vi "RT Engine.vi"(8 "Error In":errorcluster) -> ()   [LabVIEW 2013]
uses:
  <vilib>/NI/STM/TCP/TCP Connection Info.ctl
  <vilib>/NI/STM/SubVIs/MetaDataElement.ctl
  <vilib>/NI/STM/Connection Manager/TCP/TCP Connection Method.ctl
  PC/Event Mode.ctl
  <vilib>/NI/STM/Connection Manager/TCP/TCP Connection Properties.ctl
  <vilib>/NI/STM/TCP/TCP Read Options.ctl
  PC/PCsend RTrecv CMD.ctl
  TypeDef/TCP Cluster.ctl
  <vilib>/NI/STM/TCP/Write Meta Data (TCP Ref).vi
  <vilib>/NI/STM/TCP/Write Meta Data (TCP Clst).vi
  <vilib>/NI/STM/TCP/Read Message (TCP).vi
  <vilib>/NI/STM/TCP/Write Message (TCP).vi
  <vilib>/NI/STM/NI STM.lvlib
panel:
  out "conn?":bool
  out "SEND conn":T1
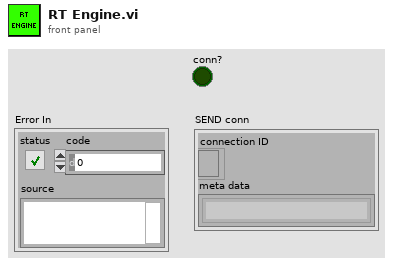
[diagram p1: front panel]
types:
  T1 = typedef "NI STM.lvlib/TCP Connection Info.ctl" = cluster{"connection ID":refnum<k5>, "meta data":T2[]}
  T2 = typedef "NI STM.lvlib/MetaDataElement.ctl" = string
  T3 = typedef "Event Mode.ctl" = enum16{"Init", "Get", "Set", "Destroy"}
  T4 = typedef "NI STM.lvlib/TCP Connection Method.ctl" = enum16{"Initialize", "Add Connection", "Set Properties", "Get Connection(s)", "Remove Connection", "Remove All Connections", "Get Connection Count"}
  T5 = typedef "NI STM.lvlib/TCP Connection Properties.ctl" = cluster{"Name":string, "Address":string, "Custom":string}
  T6 = typedef "NI STM.lvlib/TCP Read Options.ctl" = cluster{"ignore timeout error":bool, "timeout ms (1000)":i32}
  T7 = typedef "PCsend RTrecv CMD.ctl" = enum16{"ConnSettings", "Connect", "CMD", "Controller", "PSenable", "ReqCalDate", "Tolerances", "Stable Trigger", "Stop", "VPLimits", "NeedleValve", "SpeedWindow", "FreezeCmdPID", "LoadFPGA"}
  T8 = typedef "TCP Cluster.ctl" = cluster{"Command":string, "FlattenedData":string}
  T9 = typedef "RTsend PCrecv CMD.ctl" = enum16{"Data", "Connected?", "CalFileDate"}
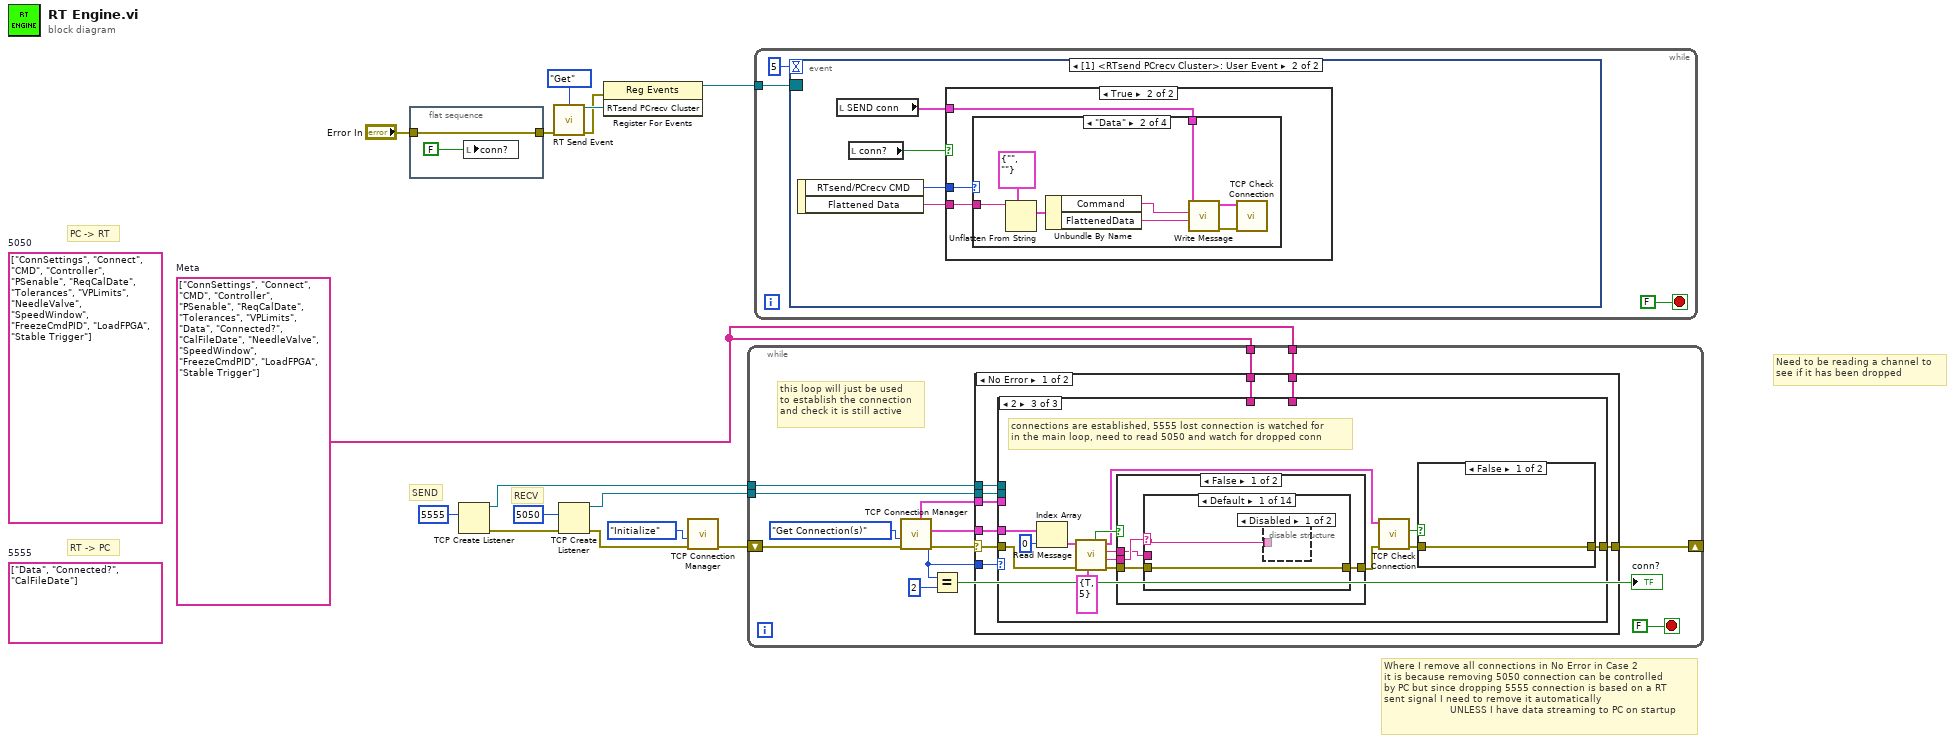
[diagram p0: block diagram]
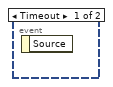
[diagram p2: hidden frame]
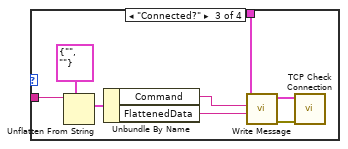
[diagram p5: hidden frame]
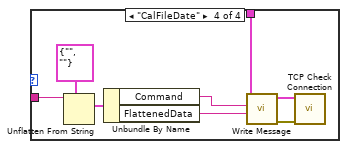
[diagram p6: hidden frame]
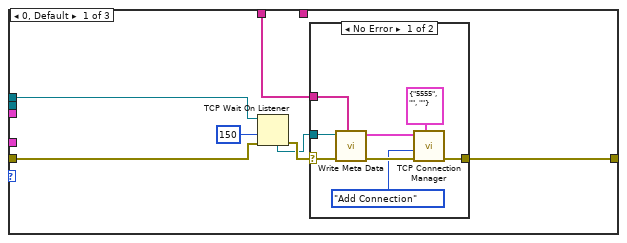
[diagram p7: hidden frame]
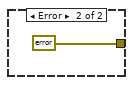
[diagram p8: hidden frame]
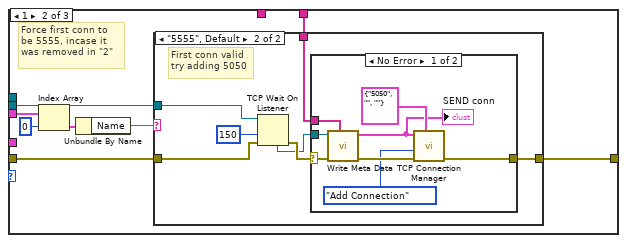
[diagram p9: hidden frame]
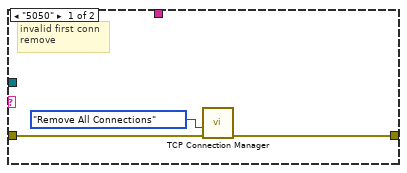
[diagram p10: hidden frame]
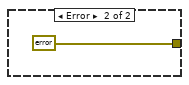
[diagram p11: hidden frame]
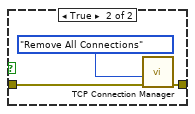
[diagram p12: hidden frame]
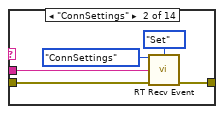
[diagram p14: hidden frame]
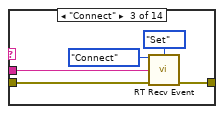
[diagram p15: hidden frame]
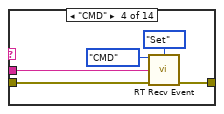
[diagram p16: hidden frame]
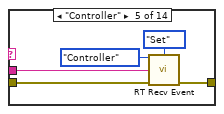
[diagram p17: hidden frame]
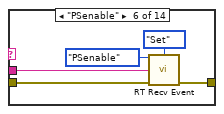
[diagram p18: hidden frame]
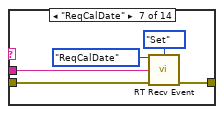
[diagram p19: hidden frame]
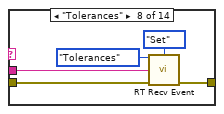
[diagram p20: hidden frame]
diagram:
  w1 = T2[] ["ConnSettings", "Connect", "CMD", "Controller", "PSenable", "ReqCalDate", "Tolerances", "VPLimits", "Data", "Connected?", "CalFileDate", "NeedleValve", "SpeedWindow", "FreezeCmdPID", "LoadFPGA", "Stable Trigger"]  # Meta
  (unwired) T2[] ["Data", "Connected?", "CalFileDate"]  # 5555
  (unwired) T2[] ["ConnSettings", "Connect", "CMD", "Controller", "PSenable", "ReqCalDate", "Tolerances", "VPLimits", "NeedleValve", "SpeedWindow", "FreezeCmdPID", "LoadFPGA", "Stable Trigger"]  # 5050
  # "PC -> RT"
  # "RT -> PC"
  # "Where I remove all connections in No Error in Case 2\nit is because removing 5050 connection can be controlled\nby PC but since dropping 5555 connection is based on a RT\nsent signal I need to remove it automatically\n                      UNLESS I have data streaming to PC on startup"
  # "Need to be reading a channel to\nsee if it has been dropped"
  # "SEND"
  # "RECV"
  n1 = flat-sequence {
    tunnel: "Error In" -> [w17]
    tunnel: [w17] -> w8
    frame #0 {
      n2 = local write "conn?"(FALSE ("stop")) -> ()
    }
  }
  n3 = TCP Create Listener(10:u16 5555 ("port")) -> (0:w6:errorcluster, 3:w5:refnum<k5>)  [unwired: 4 in, 1 out]
  n4 = call "RT Send Event.vi"("Mode"=Event_Mode."Get", "Error In"=w8) -> ("RTsend PCrecv Cluster"=w12:refnum<user-event>, "Error Out"=w11:errorcluster)  [unwired: 12 in]
  n5 = TCP Create Listener(8:w6, 10:u16 5050 ("port")) -> (0:w15:errorcluster, 3:w4:refnum<k5>)  [unwired: 3 in, 1 out]
  n6 = register-events(error in=w11, w12) -> (reference out=w10:refnum<event-registration>)  [unwired: 1 in, 1 out]
  n7 = call <vilib>:"TCP Connection Manager.vi"("error in"=w15, "method"=TCP_Connection_Method."Initialize") -> ("error out"=w13:errorcluster)  [unwired: 4 in, 5 out]
  n8 = while {
    shift-right: [w19] -> _
    shift-left: w13 -> [w31]
    tunnel: w1 -> [w28]
    tunnel: w5 -> [w25]
    tunnel: w4 -> [w24]
    tunnel: w1 -> [w18]
    stop <- FALSE stop-if-true
    # "this loop will just be used\nto establish the connection\nand check it is still active"
    n9 = call <vilib>:"TCP Connection Manager.vi"("error in"=w31, "method"=TCP_Connection_Method."Get Connection(s)") -> ("error out"=w29:errorcluster, "number of connections"=w21:i32, "all connections"=w23:T1[], "all properties"=w22:T5[])  [unwired: 4 in, 2 out]
    n10 = Equal?(x=w21, y=2) -> (x = y?=→"conn?":bool)
    n11 = case shown="No Error" w29 {
      selector: w29 -> [w40 _]
      tunnel: [w39 errorcluster {"status"=FALSE, "code"=0, "source"=""} ("t")] -> w19
      tunnel: w28 -> [w38 _]
      tunnel: w25 -> [w37 _]
      tunnel: w24 -> [w36 _]
      tunnel: w23 -> [w33 w176]
      tunnel: w22 -> [w34 _]
      tunnel: w21 -> [w35 _]
      tunnel: w18 -> [w32 _]
      frame No Error {
        n12 = case shown="2" w35 {
          tunnel: [w46 w64 w94] -> w39
          tunnel: w40 -> [w47 w57 w95]
          tunnel: w38 -> [_ w63 _]
          tunnel: w37 -> [w45 _ _]
          tunnel: w36 -> [_ w58 _]
          tunnel: w34 -> [_ w62 _]
          tunnel: w33 -> [_ _ w97]
          tunnel: w32 -> [w41 _ _]
          frame 0, Default {
            n13 = TCP Wait On Listener(8:w47, 9:150 ("timeout ms (wait forever: -1)"), 11:w45) -> (0:w43:errorcluster, 4:w42:refnum<k5>)  [unwired: 1 in, 3 out]
            n14 = case shown="No Error" w43 {
              selector: w43 -> [w55 _]
              tunnel: [w53 errorcluster {"status"=FALSE, "code"=0, "source"=""} ("error constant")] -> w46
              tunnel: w42 -> [w52 _]
              tunnel: w41 -> [w50 _]
              frame No Error {
                n15 = call-poly <vilib>:"Write Meta Data.vi"("meta data"=w50, "error in"=w55, "connection ID"=w52) -> ("error out"=w54:errorcluster, "connection info out"=w48:T1)  [unwired: 7 in]
                n16 = call <vilib>:"TCP Connection Manager.vi"("properties in"=T5 {"Name"="5555", "Address"="", "Custom"=""}, "error in"=w54, "method"=TCP_Connection_Method."Add Connection", "connection in"=w48) -> ("error out"=w53:errorcluster)  [unwired: 2 in, 5 out]
              }
              frame Error {
              }
            }
          }
          frame 1 {
            # "Force first conn to\nbe 5555, incase it\nwas removed in \"2\""
            n17 = Index Array(array=w62, index=0) -> (element=w61:T5)
            n18 = Unbundle By Name(w61) -> ("Name"=w59:string)
            n19 = case shown="\"5555\", Default" w59 {
              tunnel: [w65 w74] -> w64
              tunnel: w63 -> [_ w73]
              tunnel: w57 -> [w66 w69]
              tunnel: w58 -> [_ w68]
              frame "5050" {
                # "invalid first conn\nremove"
                n20 = call <vilib>:"TCP Connection Manager.vi"("error in"=w66, "method"=TCP_Connection_Method."Remove All Connections") -> ("error out"=w65:errorcluster)  [unwired: 4 in, 5 out]
              }
              frame "5555", Default {
                # "First conn valid\ntry adding 5050"
                n21 = TCP Wait On Listener(8:w69, 9:150 ("timeout ms (wait forever: -1)"), 11:w68) -> (0:w71:errorcluster, 4:w70:refnum<k5>)  [unwired: 1 in, 3 out]
                n22 = case shown="No Error" w71 {
                  selector: w71 -> [w82 _]
                  tunnel: [w80 errorcluster {"status"=FALSE, "code"=0, "source"=""} ("error constant")] -> w74
                  tunnel: w70 -> [w79 _]
                  tunnel: w73 -> [w77 _]
                  frame No Error {
                    n23 = call-poly <vilib>:"Write Meta Data.vi"("meta data"=w77, "error in"=w82, "connection ID"=w79) -> ("error out"=w81:errorcluster, "connection info out"=w75:T1)  [unwired: 7 in]
                    "SEND conn" <- w75
                    n24 = call <vilib>:"TCP Connection Manager.vi"("properties in"=T5 {"Name"="5050", "Address"="", "Custom"=""}, "error in"=w81, "method"=TCP_Connection_Method."Add Connection", "connection in"=w75) -> ("error out"=w80:errorcluster)  [unwired: 2 in, 5 out]
                  }
                  frame Error {
                  }
                }
              }
            }
          }
          frame 2 {
            # "connections are established, 5555 lost connection is watched for\nin the main loop, need to read 5050 and watch for dropped conn"
            n25 = Index Array(array=w97, index=0) -> (element=w93:T1)
            n26 = call-poly <vilib>:"Read Message.vi"("options"=T6 {"ignore timeout error"=TRUE, "timeout ms (1000)"=5}, "error in"=w95, "connection info in"=w93) -> ("error out"=w91:errorcluster, "name"=w90:T2, "data string"=w89:string, "connection info out"=w88:T1, "timed out?"=w92:bool)  [unwired: 3 in, 1 out]
            n27 = case shown="False" w92 {
              tunnel: w91 -> [w104 w173]
              tunnel: [w103 w173] -> w87
              tunnel: w90 -> [w105 _]
              tunnel: w89 -> [w102 _]
              frame False {
                n28 = case shown="Default" w105 {
                  selector: w105 -> [w106 _ _ _ _ _ _ _ _ _ _ _ _ _]
                  tunnel: w104 -> [w107 w111 w116 w121 w126 w131 w136 w141 w146 w151 w156 w161 w166 w171]
                  tunnel: [w107 w110 w114 w120 w125 w129 w135 w139 w144 w149 w154 w159 w164 w169] -> w103
                  tunnel: w102 -> [_ w109 w115 w119 w124 w130 w134 w140 w145 w150 w155 w160 w165 w170]
                  frame Default {
                    n29 = disable-structure shown="Disabled" {
                      disable-tunnel: w106 -> [_ _]
                      frame Disabled {
                      }
                      frame Enabled {
                      }
                    }
                  }
                  frame "ConnSettings" {
                    n30 = call "RT Recv Event.vi"("PCsend/RTrecv CMD"=PCsend_RTrecv_CMD."ConnSettings", "Mode"=Event_Mode."Set", "Flattened Data"=w109, "Error In"=w111) -> ("Error Out"=w110:errorcluster)  [unwired: 10 in, 1 out]
                  }
                  frame "Connect" {
                    n31 = call "RT Recv Event.vi"("PCsend/RTrecv CMD"=PCsend_RTrecv_CMD."Connect", "Mode"=Event_Mode."Set", "Flattened Data"=w115, "Error In"=w116) -> ("Error Out"=w114:errorcluster)  [unwired: 10 in, 1 out]
                  }
                  frame "CMD" {
                    n32 = call "RT Recv Event.vi"("PCsend/RTrecv CMD"=PCsend_RTrecv_CMD."CMD", "Mode"=Event_Mode."Set", "Flattened Data"=w119, "Error In"=w121) -> ("Error Out"=w120:errorcluster)  [unwired: 10 in, 1 out]
                  }
                  frame "Controller" {
                    n33 = call "RT Recv Event.vi"("PCsend/RTrecv CMD"=PCsend_RTrecv_CMD."Controller", "Mode"=Event_Mode."Set", "Flattened Data"=w124, "Error In"=w126) -> ("Error Out"=w125:errorcluster)  [unwired: 10 in, 1 out]
                  }
                  frame "PSenable" {
                    n34 = call "RT Recv Event.vi"("PCsend/RTrecv CMD"=PCsend_RTrecv_CMD."PSenable", "Mode"=Event_Mode."Set", "Flattened Data"=w130, "Error In"=w131) -> ("Error Out"=w129:errorcluster)  [unwired: 10 in, 1 out]
                  }
                  frame "ReqCalDate" {
                    n35 = call "RT Recv Event.vi"("PCsend/RTrecv CMD"=PCsend_RTrecv_CMD."ReqCalDate", "Mode"=Event_Mode."Set", "Flattened Data"=w134, "Error In"=w136) -> ("Error Out"=w135:errorcluster)  [unwired: 10 in, 1 out]
                  }
                  frame "Tolerances" {
                    n36 = call "RT Recv Event.vi"("PCsend/RTrecv CMD"=PCsend_RTrecv_CMD."Tolerances", "Mode"=Event_Mode."Set", "Flattened Data"=w140, "Error In"=w141) -> ("Error Out"=w139:errorcluster)  [unwired: 10 in, 1 out]
                  }
                  frame "Stable Trigger" {
                    n37 = call "RT Recv Event.vi"("PCsend/RTrecv CMD"=PCsend_RTrecv_CMD."Stable Trigger", "Mode"=Event_Mode."Set", "Flattened Data"=w145, "Error In"=w146) -> ("Error Out"=w144:errorcluster)  [unwired: 10 in, 1 out]
                  }
                  frame "VPLimits" {
                    n38 = call "RT Recv Event.vi"("PCsend/RTrecv CMD"=PCsend_RTrecv_CMD."VPLimits", "Mode"=Event_Mode."Set", "Flattened Data"=w150, "Error In"=w151) -> ("Error Out"=w149:errorcluster)  [unwired: 10 in, 1 out]
                  }
                  frame "NeedleValve" {
                    n39 = call "RT Recv Event.vi"("PCsend/RTrecv CMD"=PCsend_RTrecv_CMD."NeedleValve", "Mode"=Event_Mode."Set", "Flattened Data"=w155, "Error In"=w156) -> ("Error Out"=w154:errorcluster)  [unwired: 10 in, 1 out]
                  }
                  frame "SpeedWindow" {
                    n40 = call "RT Recv Event.vi"("PCsend/RTrecv CMD"=PCsend_RTrecv_CMD."SpeedWindow", "Mode"=Event_Mode."Set", "Flattened Data"=w160, "Error In"=w161) -> ("Error Out"=w159:errorcluster)  [unwired: 10 in, 1 out]
                  }
                  frame "FreezeCmdPID" {
                    n41 = call "RT Recv Event.vi"("PCsend/RTrecv CMD"=PCsend_RTrecv_CMD."FreezeCmdPID", "Mode"=Event_Mode."Set", "Flattened Data"=w165, "Error In"=w166) -> ("Error Out"=w164:errorcluster)  [unwired: 10 in, 1 out]
                  }
                  frame "LoadFPGA" {
                    n42 = call "RT Recv Event.vi"("PCsend/RTrecv CMD"=PCsend_RTrecv_CMD."LoadFPGA", "Mode"=Event_Mode."Set", "Flattened Data"=w170, "Error In"=w171) -> ("Error Out"=w169:errorcluster)  [unwired: 10 in, 1 out]
                  }
                }
              }
              frame True {
              }
            }
            n43 = call <vilib>:"TCP Check Connection.vi"("error in"=w87, "connection in"=w88) -> ("error out"=w86:errorcluster, "disconnected?"=w85:bool)  [unwired: 7 in, 1 out]
            n44 = case shown="False" w85 {
              tunnel: w86 -> [w98 w100]
              tunnel: [w98 w99] -> w94
              frame False {
              }
              frame True {
                n45 = call <vilib>:"TCP Connection Manager.vi"("error in"=w100, "method"=TCP_Connection_Method."Remove All Connections") -> ("error out"=w99:errorcluster)  [unwired: 4 in, 5 out]
              }
            }
          }
        }
      }
      frame Error {
        n46 = for {
          tunnel: w176 -> [w180] mode=indexing
          tunnel: errorcluster {"status"=FALSE, "code"=0, "source"=""} ("t") -> [w179]
          tunnel: [w178] -> w174
          n47 = call <vilib>:"TCP Check Connection.vi"("error in"=w179, "connection in"=w180) -> ("error out"=w178:errorcluster)  [unwired: 7 in, 2 out]
        }
        n48 = call <vilib>:"Clear Errors.vi"("error in (no error)"=w174) -> ()  [unwired: 6 in, 1 out]
      }
    }
  }
  n49 = while {
    tunnel: w10 -> [w182]
    stop <- FALSE stop-if-true
    n50 = event shown="[1] <RTsend PCrecv Cluster>: User Event" {
      selector: w182 -> [_ _]
      dyn-events: _ -> [_ _]
      timeout: 5 -> [_ _]
      event Timeout {
        n51 = event-data() -> ()  [unwired: 1 in, 1 out]
      }
      event User Event {
        n52 = event-data() -> ("RTsend/PCrecv CMD"=w185:T9, "Flattened Data"=w187:string)  [unwired: 1 in]
        n53 = local read "SEND conn"() -> (w184:T1)
        n54 = local read "conn?"() -> (w186:bool)
        n55 = case shown="True" w186 {
          tunnel: w187 -> [_ w189]
          tunnel: w185 -> [_ w190]
          tunnel: w184 -> [_ w188]
          frame False {
          }
          frame True {
            n56 = case shown="\"Data\"" w190 {
              tunnel: w188 -> [_ w194 w202 w210]
              tunnel: w189 -> [_ w193 w201 w209]
              frame Default {
              }
              frame "Data" {
                n57 = Unflatten From String(type=T8 {"Command"="", "FlattenedData"=""}, binary string=w193) -> (value=w196:T8)  [unwired: 3 in, 2 out]
                n58 = Unbundle By Name(w196) -> ("Command"=w198:string, "FlattenedData"=w197:string)
                n59 = call-poly <vilib>:"Write Message.vi"("data"=w197, "name"=w198, "connection info in"=w194) -> ("error out"=w192:errorcluster, "connection info out"=w191:T1)  [unwired: 7 in]
                n60 = call <vilib>:"TCP Check Connection.vi"("error in"=w192, "connection in"=w191) -> ()  [unwired: 7 in, 3 out]
              }
              frame "Connected?" {
                n61 = Unflatten From String(type=T8 {"Command"="", "FlattenedData"=""}, binary string=w201) -> (value=w204:T8)  [unwired: 3 in, 2 out]
                n62 = Unbundle By Name(w204) -> ("Command"=w206:string, "FlattenedData"=w205:string)
                n63 = call-poly <vilib>:"Write Message.vi"("data"=w205, "name"=w206, "connection info in"=w202) -> ("error out"=w199:errorcluster, "connection info out"=w200:T1)  [unwired: 7 in]
                n64 = call <vilib>:"TCP Check Connection.vi"("error in"=w199, "connection in"=w200) -> ()  [unwired: 7 in, 3 out]
              }
              frame "CalFileDate" {
                n65 = Unflatten From String(type=T8 {"Command"="", "FlattenedData"=""}, binary string=w209) -> (value=w212:T8)  [unwired: 3 in, 2 out]
                n66 = Unbundle By Name(w212) -> ("Command"=w214:string, "FlattenedData"=w213:string)
                n67 = call-poly <vilib>:"Write Message.vi"("data"=w213, "name"=w214, "connection info in"=w210) -> ("error out"=w207:errorcluster, "connection info out"=w208:T1)  [unwired: 7 in]
                n68 = call <vilib>:"TCP Check Connection.vi"("error in"=w207, "connection in"=w208) -> ()  [unwired: 7 in, 3 out]
              }
            }
          }
        }
      }
    }
  }
